vi "EventLoop.Queue.vi"(0 "Ctrls":refnum<vi>[](array[refnum]), 1 "Name":string, 2 "Path":path) -> ()   [LabVIEW 2014]
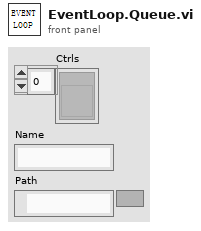
[diagram p1: front panel]
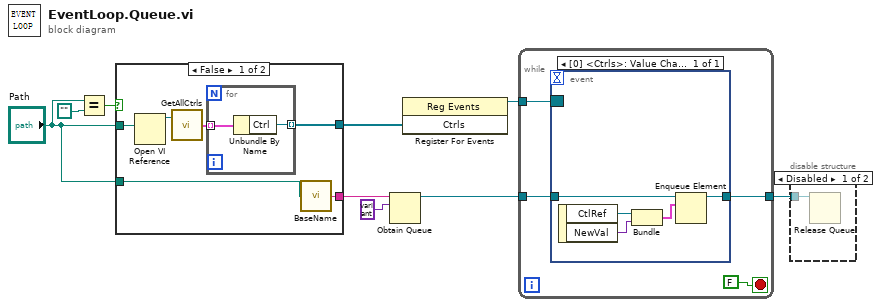
[diagram p0: block diagram]
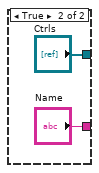
[diagram p2: hidden frame]
diagram:
  n1 = Equal?(x="Path", y=path "") -> (x = y?=w4:bool)
  n2 = case shown="False" w4 {
    tunnel: [w12 "Ctrls"] -> w3
    tunnel: [w11 "Name"] -> w2
    tunnel: "Path" -> [w13 _]
    tunnel: "Path" -> [w10 _]
    frame False {
      n3 = Open VI Reference(vi path=w13) -> (vi reference=w14:refnum<vi>)  [unwired: 5 in, 1 out]
      n4 = call "GetAllCtrls.vi"("VI"=w14) -> ("Ctrls"=w15:cluster{"Name":string, "Ctrl":refnum<vi>}[])  [unwired: 1 in]
      n5 = for {
        tunnel: w15 -> [w17] mode=indexing
        tunnel: [w16] -> w12 mode=indexing
        n6 = Unbundle By Name(w17) -> ("Ctrl"=w16:refnum<vi>)
      }
      n7 = call "BaseName.vi"("Path"=w10) -> ("Name"=w11:string)
    }
    frame True {
    }
  }
  n8 = Obtain Queue(name (unnamed)=w2, element data type=variant) -> (queue out=w7:refnum<queue>)  [unwired: 3 in, 2 out]
  n9 = register-events(w3) -> (reference out=w9:refnum<event-registration>)  [unwired: 2 in, 1 out]
  n10 = while {
    tunnel: w7 -> [w22]
    tunnel: w9 -> [w21]
    tunnel: [w20] -> w6
    stop <- FALSE stop-if-true
    n11 = event shown="[0] <Ctrls>: Value Change" {
      selector: w21 -> [_]
      dyn-events: _ -> [_]
      timeout: _ -> [_]
      tunnel: w22 -> [w28]
      tunnel: [w25] -> w20
      event Value Change {
        n12 = event-data() -> ("CtlRef"=w24:refnum<vi>, "NewVal"=w27:variant)  [unwired: 1 in]
        n13 = Bundle("CtlRef"=w24, "NewVal"=w27) -> (w26:cluster{"CtlRef":refnum<vi>, "NewVal":variant})  [unwired: 1 in]
        n14 = Enqueue Element(queue=w28, element=w26) -> (queue out=w25:refnum<queue>)  [unwired: 2 in, 2 out]
      }
    }
  }
  n15 = disable-structure shown="Disabled" {
    disable-tunnel: w6 -> [w29 _]
    frame Disabled {
      n16 = Release Queue(queue=w29) -> ()  [unwired: 2 in, 3 out]
    }
    frame Enabled {
    }
  }
